vi "getElements.vi"(8 "error in (no error)":errorcluster, 11 "tBSONDocument in":refnum<class "tBSONDocument.lvclass">) -> (0 "error out":errorcluster, 2 "Elements":refnum<class "tBSONElement.lvclass">[](array[class]), 3 "tBSONDocument out":refnum<class "tBSONDocument.lvclass">)   [LabVIEW 2013, in "BSON.lvlib" / "tBSONDocument.lvclass"]
doc: "The elements in this BSON document."
uses:
  tBSONDocument.lvclass
  tBSONElement/tBSONElement.lvclass
  tBSONDocument.lvclass/tBSONDocument.ctl
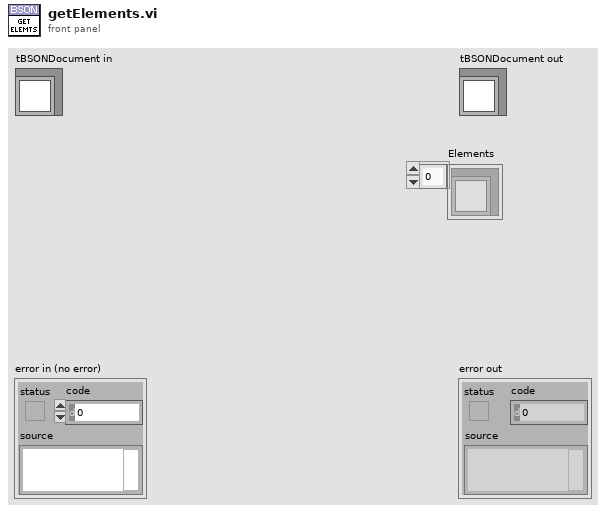
[diagram p1: front panel]
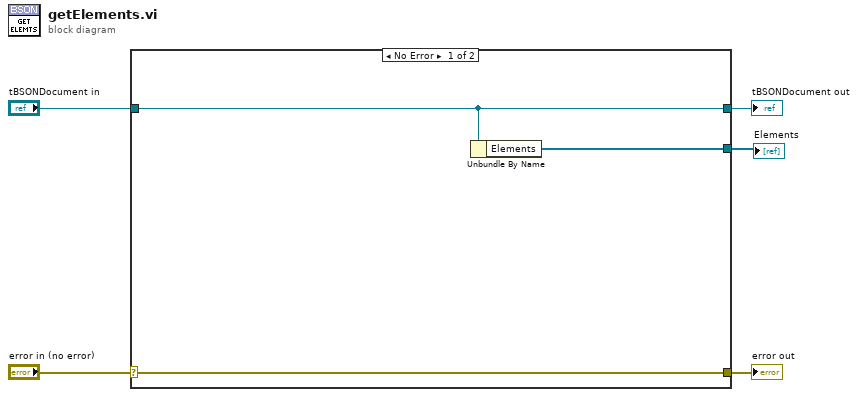
[diagram p0: block diagram]
diagram:
  n1 = case shown="No Error" "error in (no error)" {
    selector: "error in (no error)" -> [w8 w10]
    tunnel: [w8 w10] -> w4
    tunnel: [w7 w9] -> w2
    tunnel: "tBSONDocument in" -> [w7 w9]
    tunnel: [w6 _] -> w1
    frame No Error {
      n2 = Unbundle By Name(w7) -> ("Elements"=w6:refnum<class "tBSONElement.lvclass">[])
    }
    frame Error {
    }
  }
  "error out" <- w4
  "tBSONDocument out" <- w2
  "Elements" <- w1
